vi "PCO_StopRecord.vi"(8 "error in (no error)":errorcluster {"code" format="%x"}, 11 "ph":u64) -> (0 "error out":errorcluster {"code" format="%x"}, 2 "ErrorMessage":i32 format="%x", 3 "ph out":u64)   [LabVIEW 2019, in "SDK.lvlib" / "RecordingControl.lvlib"]
doc: "<b>Description:</b>\nThis function does generate a stop event for the record stop event mode. See also PCO_GetRecordStopEvent and PCO_SetRecordStopEvent.\nDue to internal timing constrains the current number of images taken after the event may differ by +/- 1 from the configured number.\n\n<b>Supported camera type:</b>\npco.1200, pco.dimax\n\n<b>Descriptor dependency:</b>\ndwGeneralCapsDESC1: RECORD_STOP"
uses:
  RecordingControl.lvlib
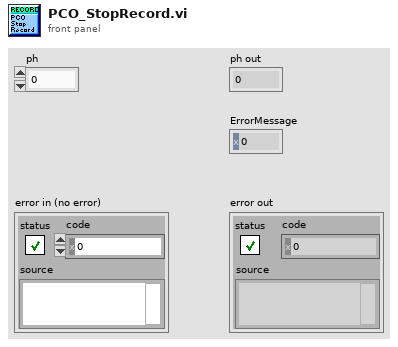
[diagram p1: front panel]
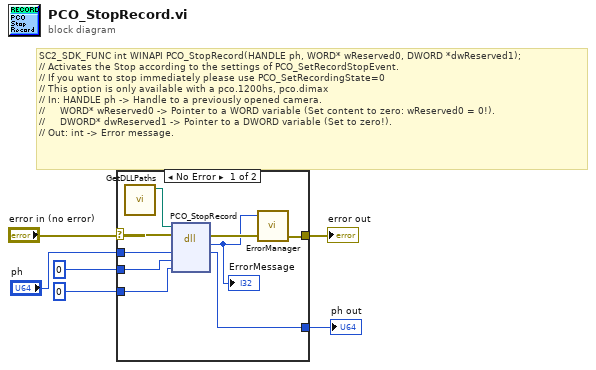
[diagram p0: block diagram]
diagram:
  # "SC2_SDK_FUNC int WINAPI PCO_StopRecord(HANDLE ph, WORD* wReserved0, DWORD *dwReserved1);\n// Activates the Stop according to the settings of PCO_SetRecordStopEvent.\n// If you want to stop immediately please use PCO_SetRecordingState=0\n// This option is only available with a pco.1200hs, pco.dimax\n// In: HANDLE ph -> Handle to a previously opened camera.\n//     WORD* wReserved0 -> Pointer to a WORD variable (Set content to zero: wReserved0 = 0!).\n//     DWORD* dwReserved1 -> Pointer to a DWORD variable (Set to zero!).\n// Out: int -> Error message."
  n1 = case shown="No Error" "error in (no error)" {
    selector: "error in (no error)" -> [w11 w17]
    tunnel: "ph" -> [w15 w16]
    tunnel: [w14 w16] -> w5
    tunnel: u16 0 ("wReserved0") -> [w13 _]
    tunnel: u32 0 ("dwReserved1") -> [w12 _]
    tunnel: [w9 w17] -> w2
    frame No Error {
      n2 = call "GetDLLPaths.vi"() -> ("SC2_Cam_Path"=w7:path)  [unwired: 8 in, 3 out]
      n3 = dll-call lib="?" fn="PCO_StopRecord"(path in=w7, error in=w11, "ph"=w15, "wReserved0"=w13, "dwReserved1"=w12) -> (error out=w10:errorcluster, "return type"=w8:i32, "ph"=w14:u64)  [unwired: 3 in, 1 out]
      "ErrorMessage" <- w8
      n4 = call "ErrorManager.vi"("error in (no error)"=w10, "error code"=w8) -> ("error out"=w9:errorcluster)  [unwired: 2 in, 1 out]
    }
    frame Error {
    }
  }
  "ph out" <- w5
  "error out" <- w2
